vi "Write configuration item.vi"(8 "error in (no error)":errorcluster, 9 "Value":string="bar", 10 "Name in":string="foo", 11 "IConfigDBQueries in":refnum<class "sqlite-queries.lvclass">) -> (0 "error out":errorcluster, 2 "Query":string="INSERT OR UPDATE INTO 'table' VALUES 'foo','bar';")   [LabVIEW 2020, in "sqlite-queries.lvlib" / "sqlite-queries.lvclass"]
uses:
  sqlite-queries.lvclass
  sqlite-queries.lvclass/sqlite-queries.ctl
  externals/database-interface/IDatabase/IDatabase.lvlib
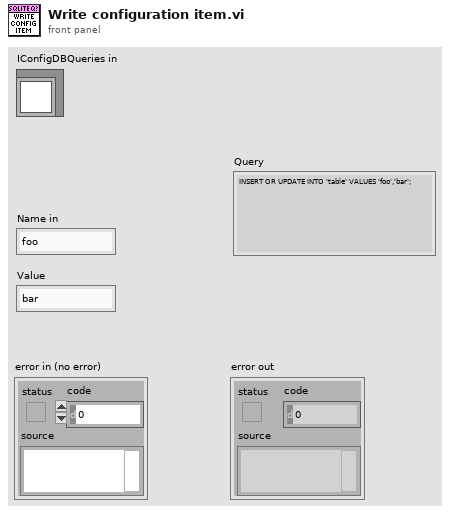
[diagram p1: front panel]
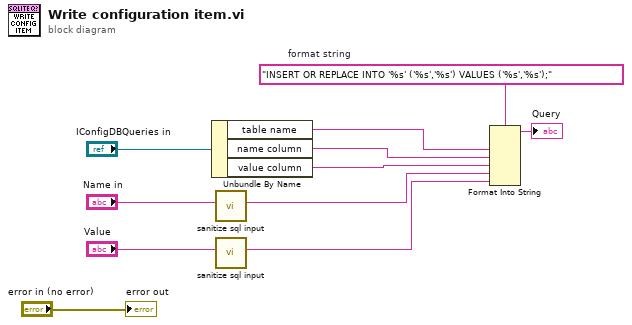
[diagram p0: block diagram]
diagram:
  w11 = "INSERT OR REPLACE INTO '%s' ('%s','%s') VALUES ('%s','%s');"  # format string
  n1 = Unbundle By Name("IConfigDBQueries in") -> ("table name"=w7:string, "name column"=w6:string, "value column"=w5:string)
  n2 = call "sanitize sql input.vi"("Sting in"="Name in") -> ("String out"=w2:string)  [unwired: 8 in, 2 out]
  n3 = call "sanitize sql input.vi"("Sting in"="Value") -> ("String out"=w1:string)  [unwired: 8 in, 2 out]
  n4 = Format Into String(format string=w11, w7, w6, w5, w2, w1) -> (resulting string=→"Query":string)  [unwired: 2 in, 1 out]
  "error out" <- "error in (no error)"
